vi "SPN.Settings.vi"(6 "Action":enum8{"Get", "Set"}(ring), 8 "error in (no error)":errorcluster, 10 "SPN.Settings":T1, 11 "Item Ref in":T2 format="%.0x") -> (0 "error out":errorcluster, 2 "SPN.Settings":T1, 3 "Item Ref out":T2 format="%.0x")   [LabVIEW 2019, in "J1939 Addon Shared.lvlib"]
uses:
  J1939 Addon Shared.lvlib
  <vilib>/NI VeriStand/Custom Device API/Custom Device Item Ref.ctl
  Types/SPN Properties.ctl
  Constants.vi
  <vilib>/NI/NI VeriStand Advanced SysDef API/_SubVIs/SysDef.Property.Set.U32.vi
  <vilib>/NI/NI VeriStand Advanced SysDef API/_SubVIs/SysDef.Property.Set.DBL.vi
  <vilib>/NI VeriStand/Custom Device API/Get Item Property (U32).vi
  <vilib>/NI VeriStand/Custom Device API/Get Item Property (Double).vi
  <vilib>/NI VeriStand/Custom Device API/Custom Device API.lvlib
  <vilib>/NI/NI VeriStand Advanced SysDef API/SysDef API/Advanced System Definition.lvlib
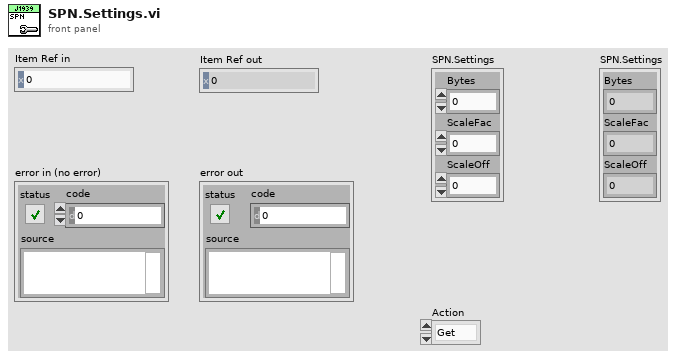
[diagram p1: front panel]
types:
  T1 = typedef "J1939 Addon Shared.lvlib/SPN Properties.ctl" = cluster{"Bytes":u32, "ScaleFac":dbl, "ScaleOff":dbl}
  T2 = typedef "Custom Device API.lvlib/Custom Device Item Ref.ctl" = u64
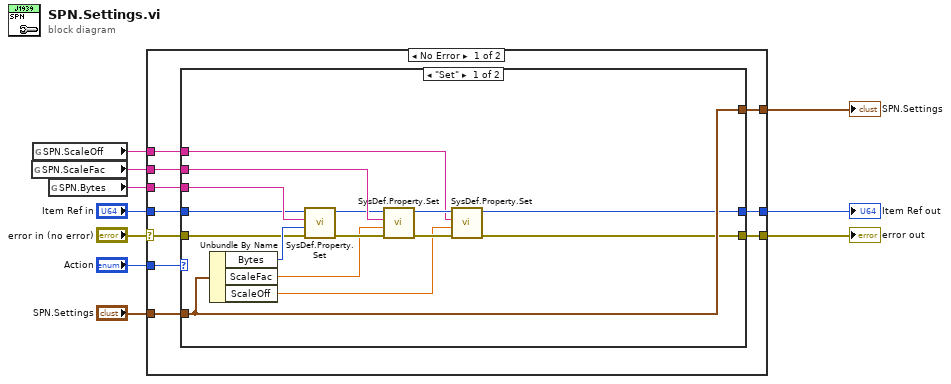
[diagram p0: block diagram]
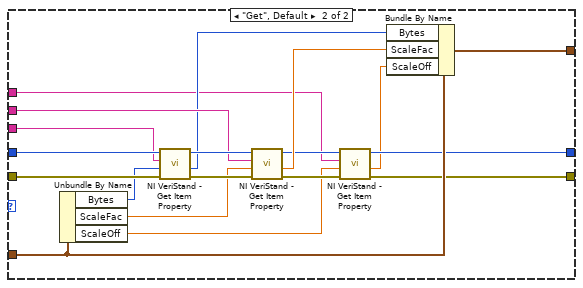
[diagram p2: hidden frame]
diagram:
  n1 = global read "Constants.vi" "SPN.ScaleFac"() -> (w5:string)
  n2 = global read "Constants.vi" "SPN.ScaleOff"() -> (w1:string)
  n3 = global read "Constants.vi" "SPN.Bytes"() -> (w9:string)
  n4 = case shown="No Error" "error in (no error)" {
    selector: "error in (no error)" -> [w14 w56]
    tunnel: "Item Ref in" -> [w20 w55]
    tunnel: w9 -> [w19 _]
    tunnel: [w18 w56] -> w8
    tunnel: [w17 w55] -> w7
    tunnel: [w16 _] -> w6
    tunnel: w5 -> [w15 _]
    tunnel: "SPN.Settings" -> [w13 _]
    tunnel: "Action" -> [w12 _]
    tunnel: w1 -> [w11 _]
    frame No Error {
      n5 = case shown="\"Set\"" w12 {
        tunnel: w20 -> [w32 w50]
        tunnel: w19 -> [w35 w47]
        tunnel: [w24 w39] -> w18
        tunnel: [w23 w40] -> w17
        tunnel: [w33 w54] -> w16
        tunnel: w15 -> [w34 w46]
        tunnel: w14 -> [w28 w51]
        tunnel: w13 -> [w33 w49]
        tunnel: w11 -> [w22 w38]
        frame "Set" {
          n6 = Unbundle By Name(w33) -> ("Bytes"=w29:u32, "ScaleFac"=w27:dbl, "ScaleOff"=w21:dbl)
          n7 = call-poly <vilib>:"SysDef.Property.Set.vi"("error in (no error)"=w28, "Value"=w29, "Property Name"=w35, "nodeID"=w32) -> ("error out"=w31:errorcluster, "nodeID out"=w30:u64)  [unwired: 6 in]
          n8 = call-poly <vilib>:"SysDef.Property.Set.vi"("error in (no error)"=w31, "Value"=w27, "Property Name"=w34, "nodeID"=w30) -> ("error out"=w25:errorcluster, "nodeID out"=w26:u64)  [unwired: 6 in]
          n9 = call-poly <vilib>:"SysDef.Property.Set.vi"("error in (no error)"=w25, "Value"=w21, "Property Name"=w22, "nodeID"=w26) -> ("error out"=w24:errorcluster, "nodeID out"=w23:u64)  [unwired: 6 in]
        }
        frame "Get", Default {
          n10 = Unbundle By Name(w49) -> ("Bytes"=w48:u32, "ScaleFac"=w44:dbl, "ScaleOff"=w36:dbl)
          n11 = call-poly <vilib>:"NI VeriStand - Get Item Property.vi"("error in (no error)"=w51, "Default Value"=w48, "Property Name"=w47, "Item Ref in"=w50) -> ("error out"=w53:errorcluster, "Value"=w45:u32, "Item Ref out"=w52:T2)  [unwired: 4 in, 1 out]
          n12 = call-poly <vilib>:"NI VeriStand - Get Item Property.vi"("error in (no error)"=w53, "Default Value"=w44, "Property Name"=w46, "Item Ref in"=w52) -> ("error out"=w41:errorcluster, "Value"=w43:dbl, "Item Ref out"=w42:T2)  [unwired: 4 in, 1 out]
          n13 = call-poly <vilib>:"NI VeriStand - Get Item Property.vi"("error in (no error)"=w41, "Default Value"=w36, "Property Name"=w38, "Item Ref in"=w42) -> ("error out"=w39:errorcluster, "Value"=w37:dbl, "Item Ref out"=w40:T2)  [unwired: 4 in, 1 out]
          n14 = Bundle By Name(cluster=w49, "Bytes"=w45, "ScaleFac"=w43, "ScaleOff"=w37) -> (w54:T1)
        }
      }
    }
    frame Error {
    }
  }
  "Item Ref out" <- w7
  "error out" <- w8
  "SPN.Settings" <- w6
